vi "zmq_version.vi"(3 "error in":errorcluster) -> (0 "error out":errorcluster, 1 "version":cluster{"major":i32, "minor":i32, "fix":i32}, 2 "version string":string)   [LabVIEW 2020, in "zeromq.lvlib"]
doc: "Queries and returns the version of ZeroMQ currently loaded as both a string and struct.\n\nDetailed API documentation: http://api.zeromq.org/3-2:zmq-version"
uses:
  zeromq.lvlib
panel:
  # "ØMQ"
  # "labview"
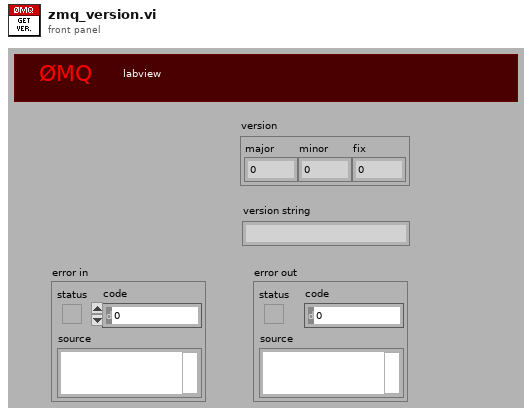
[diagram p1: front panel]
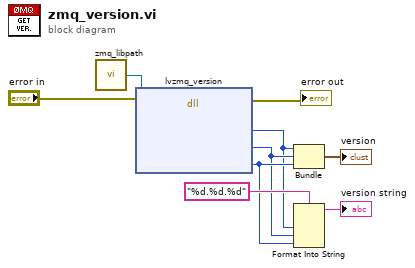
[diagram p0: block diagram]
diagram:
  n1 = call "zmq_libpath.vi"() -> ("path"=w1:path)
  n2 = dll-call lib="?" fn="lvzmq_version" ("zmq_labview.dll:lvzmq_socket")(path in=w1, error in="error in") -> (error out=→"error out":errorcluster, "maj"=w4:i32, "min"=w5:i32, "fix"=w6:i32)  [unwired: 5 in, 1 out]
  n3 = Bundle("maj"=w4, "min"=w5, "fix"=w6) -> (→"version":cluster{"maj":i32, "min":i32, "fix":i32})  [unwired: 1 in]
  n4 = Format Into String(format string="%d.%d.%d", w4, w5, w6) -> (resulting string=→"version string":string)  [unwired: 2 in, 1 out]
